vi "Calculate Current Magnitude Measurements.vi"(8 "Voltage Waveform":dbl[](array[numeric]), 9 "Current Waveform":dbl[](array[numeric]), 10 "Event.Parameters":T1={"Shots"=0, "Shot.InitialVoltage"=0.0, "Shot.Stages"=0, "Stages"=[{"Stage.Dwell.Level"=0.0, "PullIn.Type"=enum."Pull In Transition Pulses", "PullIn.Level"=0.0, "Transition.Type"=enum."Stage Transition Voltage Increase", "Transition.Level"=0.0, "Results"={"Pull In Time"=TRUE, "Pull In Max Current"=TRUE, "Pull In Max Voltage"=TRUE, "Pull In Min Voltage"=TRUE, "Pull In Avg Voltage"=TRUE, "Hold Time"=TRUE, "Hold Max Current"=TRUE, "Hold Min Current"=TRUE, "Hold Avg Current"=TRUE, "Hold Max Voltage"=TRUE, "Hold Min Voltage"=TRUE, "Hold Avg Max Voltage"=TRUE, "Hold Avg Min Voltage"=TRUE, "Off Time"=TRUE, "Off Max Current"=TRUE, "Off Min Current"=TRUE, "Off Avg Current"=TRUE, "Off Max Voltage"=TRUE, "Off Min Voltage"=TRUE, "Off Avg Voltage"=TRUE, "Total Voltage Pulses"=TRUE, "Total Stage Time"=TRUE}}], "Timeout"=0.0, "Results.Count"=0, "Active Edge"=FALSE, "Rate.Hz"=0, "Channels"=0}, 11 "Shot Info Array":T6[](array[typedef]) {"Results"."Off-Stage Min Volt" format="%#.6g"; "Results"."Off-Stage Avg Volt" format="%#.6g"; "Results"."Off-Stage Max Volt" format="%#.6g"; "Results"."Total Stage Time (us)" format="%#.6g"; "Results"."Off-Stage Avg Current" format="%#.6g"; "Results"."Total Voltage Pulses" format="%#.6g"; "Results"."Off-Stage Min Current" format="%#.6g"; "Results"."Off-Stage Max Current" format="%#.6g"}) -> (3 "Shot Info Array":T6[](array[typedef]) {"Results"."Off-Stage Min Volt" format="%#.6g"; "Results"."Off-Stage Avg Volt" format="%#.6g"; "Results"."Off-Stage Max Volt" format="%#.6g"; "Results"."Total Stage Time (us)" format="%#.6g"; "Results"."Off-Stage Avg Current" format="%#.6g"; "Results"."Total Voltage Pulses" format="%#.6g"; "Results"."Off-Stage Min Current" format="%#.6g"; "Results"."Off-Stage Max Current" format="%#.6g"})   [LabVIEW 2019, in "Fuel Injector Analysis Addon Engine.lvlib"]
uses:
  Fuel Injector Analysis Addon Engine.lvlib
  Controls/Shot Information Control.ctl
  Types/Stage.Measurements.ctl
  Addon Shared/Types/Shot.Parameters.ctl
  Addon Shared/Types/Stage.Parameters.ctl
  Addon Shared/Types/Stage.PullIn.Types.ctl
  Addon Shared/Types/Stage.Transition.Types.ctl
  Addon Shared/Types/Analysis.Channels.Select.ctl
  <vilib>/Analysis/baseanly.llb/Mean (DBL).vi
  Addon Shared/Constants.vi
  Addon Shared/Fuel Injector Analysis Addon Shared.lvlib
  <vilib>/Analysis/NI_AALBase.lvlib
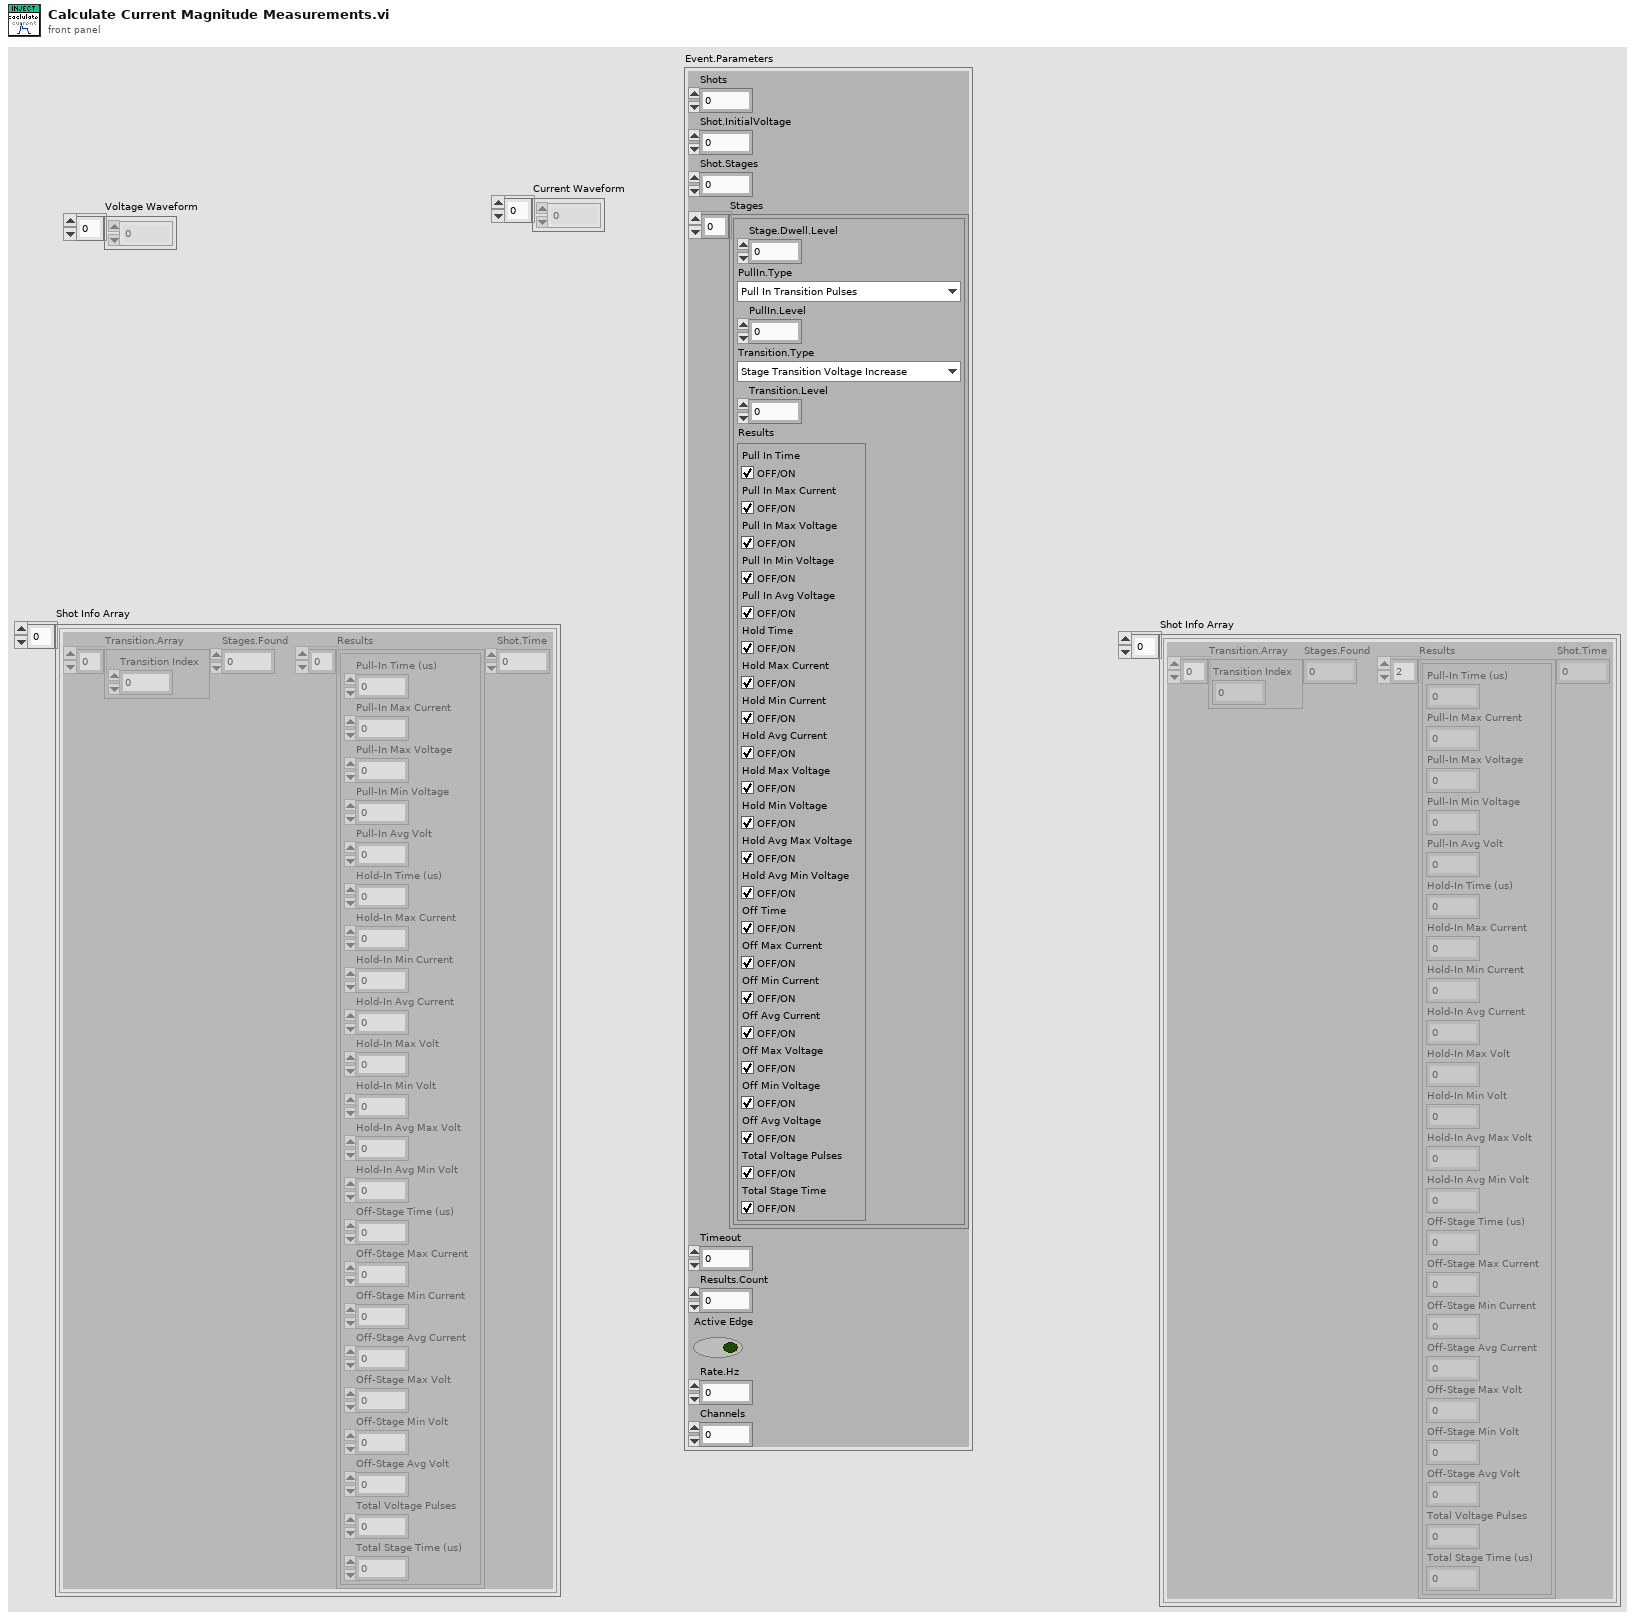
[diagram p1: front panel]
types:
  T1 = typedef "Fuel Injector Analysis Addon Shared.lvlib/Shot.Parameters.ctl" = cluster{"Shots":u32, "Shot.InitialVoltage":dbl, "Shot.Stages":u32, "Stages":T2[], "Timeout":dbl, "Results.Count":i32, "Active Edge":bool, "Rate.Hz":u32, "Channels":u32}
  T2 = typedef "Fuel Injector Analysis Addon Shared.lvlib/Stage.Parameters.ctl" = cluster{"Stage.Dwell.Level":dbl, "PullIn.Type":T3, "PullIn.Level":dbl, "Transition.Type":T4, "Transition.Level":dbl, "Results":T5}
  T3 = typedef "Fuel Injector Analysis Addon Shared.lvlib/Stage.PullIn.Types.ctl" = enum8{"Pull In Transition Pulses", "Pull In Transition Current Drop"}
  T4 = typedef "Fuel Injector Analysis Addon Shared.lvlib/Stage.Transition.Types.ctl" = enum8{"Stage Transition Inactive Time", "Stage Transition Voltage Increase", "Stage Transition Current Decrease", "Stage Transition Active Time"}
  T5 = typedef "Fuel Injector Analysis Addon Shared.lvlib/Analysis.Channels.Select.ctl" = cluster{"Pull In Time":bool, "Pull In Max Current":bool, "Pull In Max Voltage":bool, "Pull In Min Voltage":bool, "Pull In Avg Voltage":bool, "Hold Time":bool, "Hold Max Current":bool, "Hold Min Current":bool, "Hold Avg Current":bool, "Hold Max Voltage":bool, "Hold Min Voltage":bool, "Hold Avg Max Voltage":bool, "Hold Avg Min Voltage":bool, "Off Time":bool, "Off Max Current":bool, "Off Min Current":bool, "Off Avg Current":bool, "Off Max Voltage":bool, "Off Min Voltage":bool, "Off Avg Voltage":bool, "Total Voltage Pulses":bool, "Total Stage Time":bool}
  T6 = typedef "Fuel Injector Analysis Addon Engine.lvlib/Shot Information Control.ctl" = cluster{"Transition.Array":i32[], "Stages.Found":u16, "Results":T7[], "Shot.Time":dbl}
  T7 = typedef "Fuel Injector Analysis Addon Engine.lvlib/Stage.Measurements.ctl" = cluster{"Pull-In Time (us)":dbl, "Pull-In Max Current":dbl, "Pull-In Max Voltage":dbl, "Pull-In Min Voltage":dbl, "Pull-In Avg Volt":dbl, "Hold-In Time (us)":dbl, "Hold-In Max Current":dbl, "Hold-In Min Current":dbl, "Hold-In Avg Current":dbl, "Hold-In Max Volt":dbl, "Hold-In Min Volt":dbl, "Hold-In Avg Max Volt":dbl, "Hold-In Avg Min Volt":dbl, "Off-Stage Time (us)":dbl, "Off-Stage Max Current":dbl, "Off-Stage Min Current":dbl, "Off-Stage Avg Current":dbl, "Off-Stage Max Volt":dbl, "Off-Stage Min Volt":dbl, "Off-Stage Avg Volt":dbl, "Total Voltage Pulses":dbl, "Total Stage Time (us)":dbl}
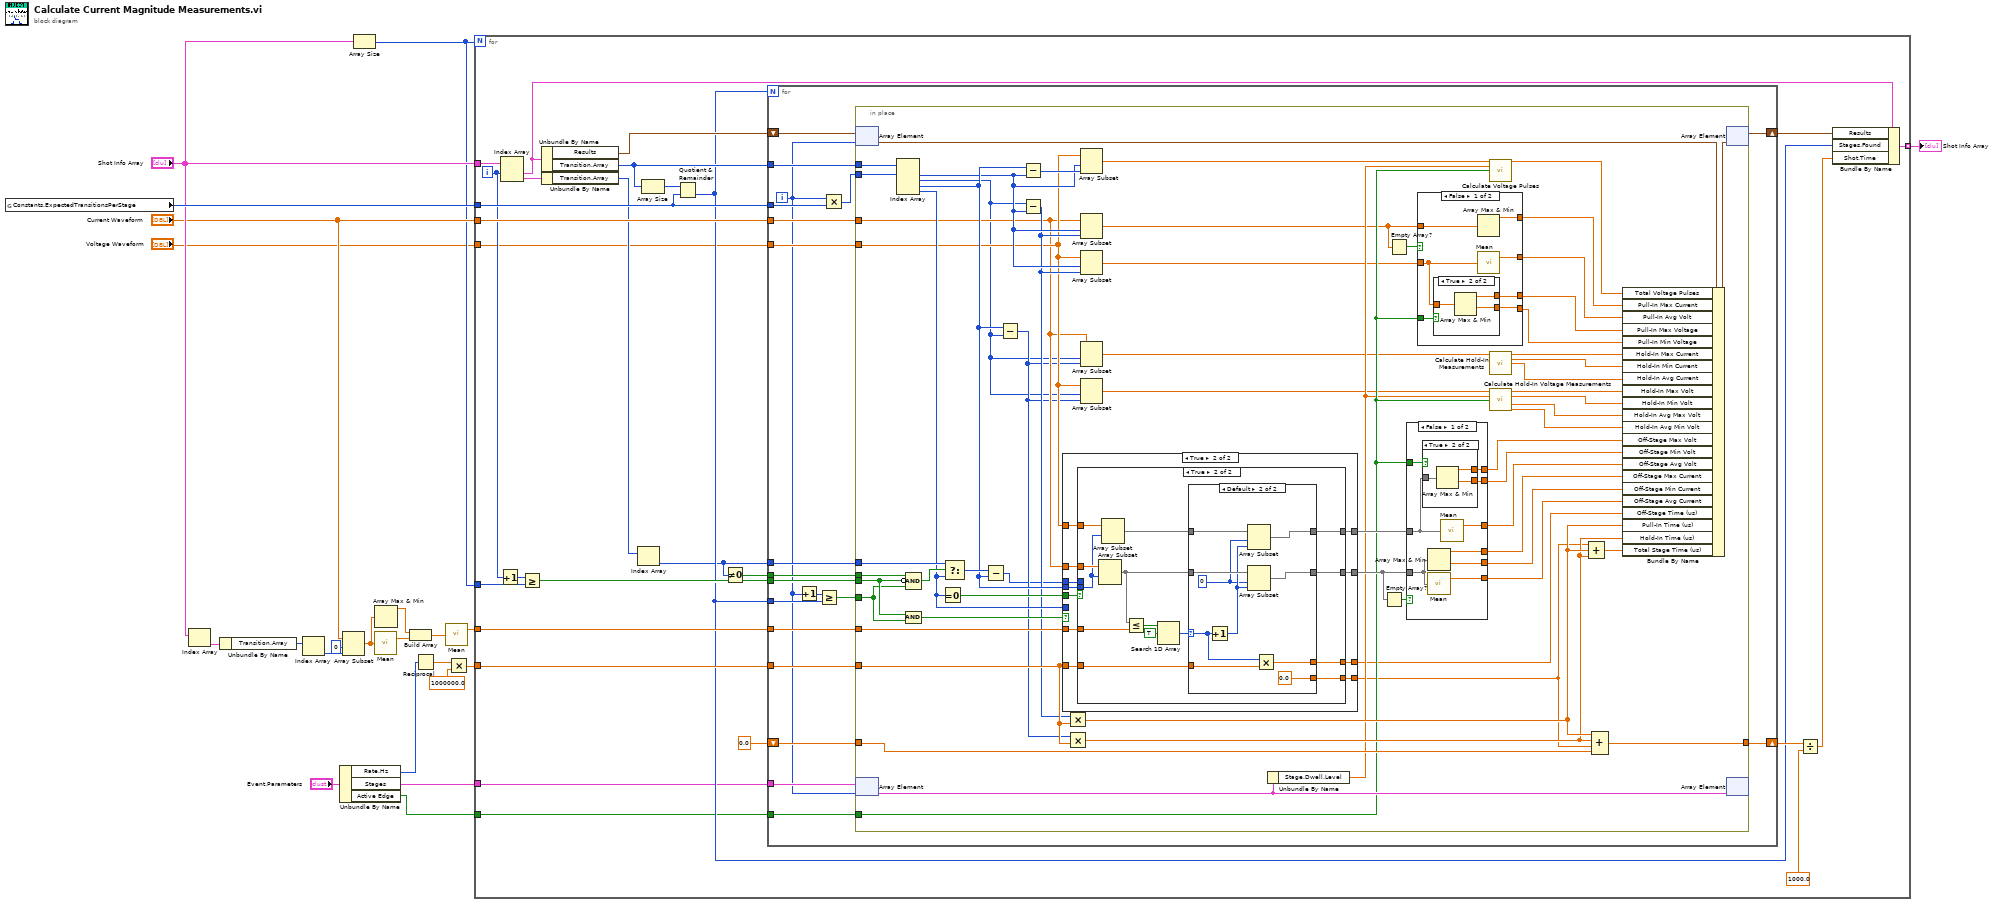
[diagram p0: block diagram]
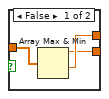
[diagram p2: hidden frame]
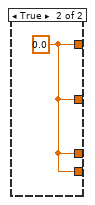
[diagram p3: hidden frame]
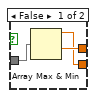
[diagram p4: hidden frame]
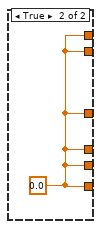
[diagram p5: hidden frame]
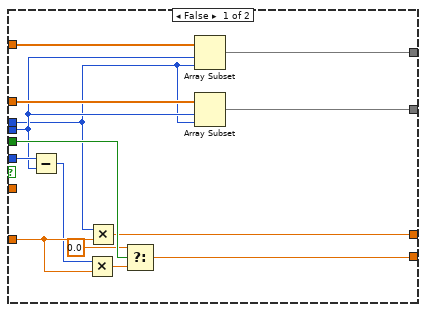
[diagram p6: hidden frame]
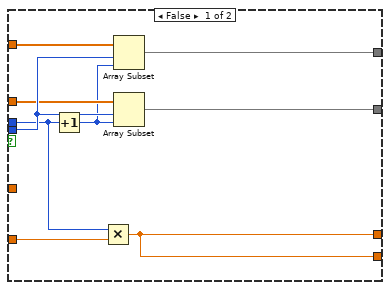
[diagram p7: hidden frame]
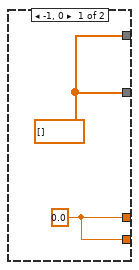
[diagram p8: hidden frame]
diagram:
  n1 = global read "Constants.vi" "Constants.ExpectedTransitionsPerStage"() -> (w21:u32)
  n2 = Index Array(array="Shot Info Array") -> (element=w16:T6)  [unwired: 1 in]
  n3 = Unbundle By Name(w16) -> ("Transition.Array"=w13:i32[])
  n4 = Index Array(array=w13) -> (element=w15:i32)  [unwired: 1 in]
  n5 = Unbundle By Name("Event.Parameters") -> ("Rate.Hz"=w1:u32, "Stages"=w3:T2[], "Active Edge"=w2:bool)
  n6 = Array Subset(array="Current Waveform", index=0, length=w15) -> (w10:dbl[])
  n7 = Array Size(array="Shot Info Array") -> (size(s)=w11:i32)
  n8 = call-poly <vilib>:"Mean.vi"("X"=w10) -> ("mean"=w7:dbl)  [unwired: 1 out]
  n9 = Array Max & Min(array=w10) -> (max value=w9:dbl)  [unwired: 3 out]
  n10 = Build Array(w9, w7) -> (w8:dbl[])
  n11 = Reciprocal(x=w1) -> (1/x=w18:dbl)
  n12 = call-poly <vilib>:"Mean.vi"("X"=w8) -> ("mean"=w6:dbl)  [unwired: 1 out]
  n13 = Multiply(x=w18, y=1000000.0) -> (x*y=w19:dbl)
  n14 = for {
    N: w11 -> [_]
    tunnel: "Current Waveform" -> [w43]
    tunnel: [w49] -> w22 mode=indexing
    tunnel: w21 -> [w45]
    tunnel: w19 -> [w44]
    tunnel: "Shot Info Array" -> [w38]
    tunnel: w6 -> [w33]
    tunnel: w11 -> [w30]
    tunnel: "Voltage Waveform" -> [w25]
    tunnel: w3 -> [w24]
    tunnel: w2 -> [w23]
    i -> [w32]
    n15 = Increment(x=w32) -> (x+1=w31:i32)
    n16 = Index Array(array=w38, index #1=w32) -> (element #1=w37:T6, element #2=w36:T6)  [unwired: 1 in]
    n17 = Greater Or Equal?(x=w31, y=w30) -> (x >= y?=w29:bool)
    n18 = Unbundle By Name(w37) -> ("Results"=w48:T7[], "Transition.Array"=w34:i32[])
    n19 = Unbundle By Name(w36) -> ("Transition.Array"=w35:i32[])
    n20 = Index Array(array=w35) -> (element=w27:i32)  [unwired: 1 in]
    n21 = Array Size(array=w34) -> (size(s)=w46:i32)
    n22 = Quotient & Remainder(x=w46, y=w45) -> (floor(x/y)=w28:u32)  [unwired: 1 out]
    n23 = Not Equal To 0?(x=w27) -> (x != 0?=w26:bool)
    n24 = for {
      N: w28 -> [_]
      tunnel: w43 -> [w69]
      tunnel: w34 -> [w65]
      shift-right: [w66] -> w47
      shift-left: w48 -> [w68]
      tunnel: w45 -> [w64]
      tunnel: w44 -> [w63]
      tunnel: w33 -> [w62]
      shift-right: [w61] -> w41
      shift-left: 0.0 -> [w60]
      tunnel: w28 -> [w59]
      tunnel: w29 -> [w57]
      tunnel: w27 -> [w56]
      tunnel: w26 -> [w54]
      tunnel: w25 -> [w53]
      tunnel: w24 -> [w52]
      tunnel: w23 -> [w50]
      i -> [w51]
      n25 = Increment(x=w51) -> (x+1=w55:i32)
      n26 = Greater Or Equal?(x=w55, y=w59) -> (x >= y?=w58:bool)
      n27 = Multiply(x=w51, y=w64) -> (x*y=w67:u32)
      n28 = in-place {
        in-place-border: w69 -> [w82]
        in-place-border: w65 -> [w130]
        in-place-border: w67 -> [w127]
        in-place-border: w63 -> [w123]
        in-place-border: w62 -> [w119]
        in-place-border: [w117] -> w61
        in-place-border: w60 -> [w116]
        in-place-border: w58 -> [w113]
        in-place-border: w57 -> [w114]
        in-place-border: w56 -> [w109]
        in-place-border: w54 -> [w108]
        in-place-border: w53 -> [w83]
        in-place-border: w50 -> [w90]
        n29 = in-place-array #1(w68, w51) -> (w126:T7)
        n30 = in-place-array #2(w52, w51) -> (w99:T2)
        n31 = Index Array(array=w130, index #1=w127) -> (element #1=w85:i32, element #2=w79:i32, element #3=w101:i32, element #4=w107:i32)  [unwired: 3 in]
        n32 = Compound Arithmetic op=AND(w108, invert w114, w113) -> (w115:bool)
        n33 = Compound Arithmetic op=AND(w114, w113) -> (w112:bool)
        n34 = Equal To 0?(x=w107) -> (x = 0?=w110:bool)
        n35 = Select(t=w109, s=w115, f=w107) -> (s? t:f=w111:i32)
        n36 = Subtract(x=w111, y=w101) -> (x-y=w70:i32)
        n37 = Subtract(x=w101, y=w79) -> (x-y=w80:i32)
        n38 = Subtract(x=w101, y=w85) -> (x-y=w86:i32)
        n39 = Subtract(x=w79, y=w85) -> (x-y=w84:i32)
        n40 = case shown="True" w112 {
          tunnel: w82 -> [w174 w185]
          tunnel: w101 -> [w164 w181]
          tunnel: w70 -> [w161 w178]
          tunnel: w123 -> [w172 w184]
          tunnel: [w173 w182] -> w103
          tunnel: w119 -> [_ w183]
          tunnel: [w162 w180] -> w71
          tunnel: w110 -> [w171 w179]
          tunnel: w107 -> [w168 _]
          tunnel: w83 -> [w166 w177]
          tunnel: [w165 w176] -> w100
          tunnel: [w163 w175] -> w72
          frame False {
            n41 = Subtract(x=w168, y=w164) -> (x-y=w167:i32)
            n42 = Multiply(x=w167, y=w172) -> (x*y=w170:dbl)
            n43 = Multiply(x=w161, y=w172) -> (x*y=w163:dbl)
            n44 = Select(t=0.0, s=w171, f=w170) -> (s? t:f=w162:dbl)
            n45 = Array Subset(array=w166, index=w164, length=w161) -> (w165:dbl[])
            n46 = Array Subset(array=w174, index=w164, length=w161) -> (w173:dbl[])
          }
          frame True {
            n47 = case shown="True" w179 {
              tunnel: w185 -> [w190 w208]
              tunnel: w184 -> [w194 w205]
              tunnel: w183 -> [_ w204]
              tunnel: [w189 w202] -> w182
              tunnel: w181 -> [w191 w197]
              tunnel: [w188 w199] -> w180
              tunnel: w178 -> [w187 _]
              tunnel: w177 -> [w192 w196]
              tunnel: [w193 w200] -> w176
              tunnel: [w188 w198] -> w175
              frame False {
                n48 = Increment(x=w187) -> (x+1=w186:i32)
                n49 = Multiply(x=w187, y=w194) -> (x*y=w188:dbl)
                n50 = Array Subset(array=w192, index=w191, length=w186) -> (w193:dbl[])
                n51 = Array Subset(array=w190, index=w191, length=w186) -> (w189:dbl[])
              }
              frame True {
                n52 = Array Subset(array=w208, index=w197) -> (w203:dbl[])  [unwired: 1 in]
                n53 = Array Subset(array=w196, index=w197) -> (w195:dbl[])  [unwired: 1 in]
                n54 = Less Or Equal?(x=w203, y=w204) -> (x <= y?=w207:bool[])
                n55 = Search 1D Array(1D array=w207, element=TRUE) -> (index of element=w201:i32)  [unwired: 1 in]
                n56 = case shown="Default" w201 {
                  selector: w201 -> [_ w213]
                  tunnel: w205 -> [_ w220]
                  tunnel: [w210 w219] -> w198
                  tunnel: w203 -> [_ w218]
                  tunnel: [w209 w217] -> w202
                  tunnel: [w210 0.0 ("x*y")] -> w199
                  tunnel: w195 -> [_ w215]
                  tunnel: [w209 w214] -> w200
                  frame -1, 0 {
                    w209 = dbl[] []
                    w210 = 0.0
                  }
                  frame Default {
                    w211 = 0 ("index")
                    n57 = Increment(x=w213) -> (x+1=w212:i32)
                    n58 = Array Subset(array=w215, index=w211, length=w212) -> (w214:dbl[])
                    n59 = Array Subset(array=w218, index=w211, length=w212) -> (w217:dbl[])
                    n60 = Multiply(x=w213, y=w220) -> (x*y=w219:dbl)
                  }
                }
              }
            }
          }
        }
        n61 = Multiply(x=w84, y=w123) -> (x*y=w106:dbl)
        n62 = Multiply(x=w80, y=w123) -> (x*y=w105:dbl)
        n63 = Array Subset(array=w83, index=w85, length=w86) -> (w87:dbl[])
        n64 = Array Subset(array=w82, index=w85, length=w84) -> (w75:dbl[])
        n65 = Array Subset(array=w83, index=w85, length=w84) -> (w77:dbl[])
        n66 = Array Subset(array=w82, index=w79, length=w80) -> (w81:dbl[])
        n67 = Array Subset(array=w83, index=w79, length=w80) -> (w78:dbl[])
        n68 = Unbundle By Name(w99) -> ("Stage.Dwell.Level"=w89:dbl)
        n69 = Empty Array?(array=w103) -> (empty?=w102:bool)
        n70 = Empty Array?(array=w75) -> (empty?=w76:bool)
        n71 = case shown="False" w102 {
          tunnel: [w153 w160] -> w122
          tunnel: [w152 w160] -> w121
          tunnel: [w151 w160] -> w120
          tunnel: w103 -> [w150 _]
          tunnel: w100 -> [w149 _]
          tunnel: [w148 w160] -> w91
          tunnel: [w147 w160] -> w88
          tunnel: w90 -> [w146 _]
          tunnel: [w145 w160] -> w74
          frame False {
            n72 = case shown="True" w146 {
              tunnel: w149 -> [w156 w159]
              tunnel: [w155 w158] -> w148
              tunnel: [w154 w157] -> w145
              frame False {
                n73 = Array Max & Min(array=w156) -> (max value=w154:dbl, min value=w155:dbl)  [unwired: 2 out]
              }
              frame True {
                n74 = Array Max & Min(array=w159) -> (max value=w158:dbl, min value=w157:dbl)  [unwired: 2 out]
              }
            }
            n75 = Array Max & Min(array=w150) -> (max value=w153:dbl, min value=w152:dbl)  [unwired: 2 out]
            n76 = call-poly <vilib>:"Mean.vi"("X"=w150) -> ("mean"=w151:dbl)  [unwired: 1 out]
            n77 = call-poly <vilib>:"Mean.vi"("X"=w149) -> ("mean"=w147:dbl)  [unwired: 1 out]
          }
          frame True {
            w160 = 0.0 ("mean")
          }
        }
        n78 = case shown="False" w76 {
          tunnel: w75 -> [w137 _]
          tunnel: [w136 w144] -> w118
          tunnel: [w135 w144] -> w98
          tunnel: [w134 w144] -> w97
          tunnel: w90 -> [w133 _]
          tunnel: w77 -> [w132 _]
          tunnel: [w131 w144] -> w73
          frame False {
            n79 = case shown="True" w133 {
              tunnel: w132 -> [w140 w143]
              tunnel: [w139 w142] -> w135
              tunnel: [w138 w141] -> w131
              frame False {
                n80 = Array Max & Min(array=w140) -> (max value=w138:dbl, min value=w139:dbl)  [unwired: 2 out]
              }
              frame True {
                n81 = Array Max & Min(array=w143) -> (max value=w142:dbl, min value=w141:dbl)  [unwired: 2 out]
              }
            }
            n82 = Array Max & Min(array=w137) -> (max value=w136:dbl)  [unwired: 3 out]
            n83 = call-poly <vilib>:"Mean.vi"("X"=w132) -> ("mean"=w134:dbl)  [unwired: 1 out]
          }
          frame True {
            w144 = 0.0
          }
        }
        n84 = call "Calculate Voltage Pulses.vi"("Stage Voltage Section"=w87, "Stage.Dwell.Level"=w89, "Active Edge"=w90) -> ("# of Pulses"=w96:dbl)  [unwired: 12 in]
        n85 = call "Calculate Hold-In Measurements.vi"("Stage Waveform Section"=w81) -> ("Max Stage"=w129:dbl, "Min Stage"=w128:dbl, "Avg Stage"=w124:dbl)  [unwired: 10 in, 2 out]
        n86 = call "Calculate Hold-In Voltage Measurements.vi"("Stage Voltage Section"=w78, "Stage.Dwell.Level"=w89, "Active Edge"=w90) -> ("Max Stage"=w95:dbl, "Min Stage"=w94:dbl, "Avg Max Stage"=w93:dbl, "Avg Min Stage"=w92:dbl)  [unwired: 9 in]
        n87 = Compound Arithmetic op=ADD(w71, w106, w105) -> (w104:dbl)
        n88 = Compound Arithmetic op=ADD(w106, w105, w71, w116) -> (w117:dbl)
        n89 = Bundle By Name(cluster=w126, "Total Voltage Pulses"=w96, "Pull-In Max Current"=w118, "Pull-In Avg Volt"=w97, "Pull-In Max Voltage"=w98, "Pull-In Min Voltage"=w73, "Hold-In Max Current"=w129, "Hold-In Min Current"=w128, "Hold-In Avg Current"=w124, "Hold-In Max Volt"=w95, "Hold-In Min Volt"=w94, "Hold-In Avg Max Volt"=w93, "Hold-In Avg Min Volt"=w92, "Off-Stage Max Volt"=w91, "Off-Stage Min Volt"=w74, "Off-Stage Avg Volt"=w88, "Off-Stage Max Current"=w122, "Off-Stage Min Current"=w121, "Off-Stage Avg Current"=w120, "Off-Stage Time (us)"=w72, "Pull-In Time (us)"=w106, "Hold-In Time (us)"=w105, "Total Stage Time (us)"=w104) -> (w125:T7)
        n90 = in-place-array #1(w125) -> (w66:T7[])  [unwired: 1 out]
        n91 = in-place-array #2(w99) -> ()  [unwired: 2 out]
      }
    }
    n92 = Divide(x=w41, y=1000.0) -> (x/y=w40:dbl)
    n93 = Bundle By Name(cluster=w37, "Results"=w47, "Stages.Found"=w28, "Shot.Time"=w40) -> (w49:T6)
  }
  "Shot Info Array" <- w22
